vi "Check.vi"(8 "error in (no error)":errorcluster) -> (0 "error out":errorcluster, 3 "Pass? ( T)":bool=TRUE)   [LabVIEW 2017, in "WebServiceImporter.lvlib" / "Main Panel.lvlib" / "Authentication.lvlib"]
uses:
  <vilib>/Platform/WebService/Main Panel/Pages/Authentication/Authentication.lvlib
  <vilib>/Platform/WebService/Main Panel/Events/Events.lvlib
  <vilib>/Platform/WebService/Main Panel/Pages/Authentication/Events/Events.lvlib
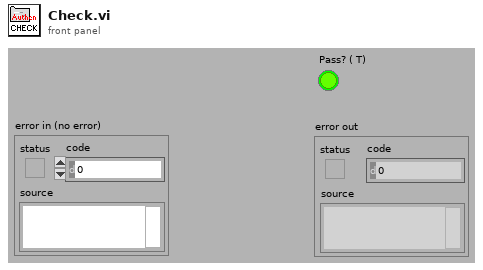
[diagram p1: front panel]
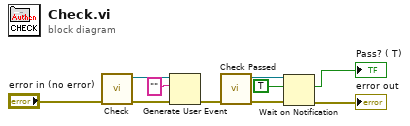
[diagram p0: block diagram]
diagram:
  n1 = call <vilib>:"Check.vi"("error in (no error)"="error in (no error)") -> ("error out"=w1:errorcluster, "user event (out)"=w2:refnum<user-event>)  [unwired: 9 in]
  n2 = Generate User Event(user event=w2, event data cluster="" ("event data"), error in=w1) -> (error out=w9:errorcluster)  [unwired: 1 in, 1 out]
  n3 = call <vilib>:"Check Passed.vi"("error in (no error)"=w9) -> ("error out"=w8:errorcluster, "notifier  (out)"=w7:refnum<notifier>)  [unwired: 9 in]
  n4 = Wait on Notification(notifier=w7, ignore previous (F)=TRUE, error in (no error)=w8) -> (notification=→"Pass? ( T)":bool, error out=→"error out":errorcluster)  [unwired: 1 in, 2 out]
